vi "Save Data (SubVI).vi"(0 "Time":dbl, 1 "Impedance":dbl[](array[numeric]), 2 "Phase":dbl[](array[numeric]), 3 "error in":errorcluster, 4 "Temperature":dbl, 5 "Byte Stream File in":refnum<file>) -> (6 "error out":errorcluster)   [LabVIEW 2017]
uses:
  GlobalVariables/Delimiter.vi
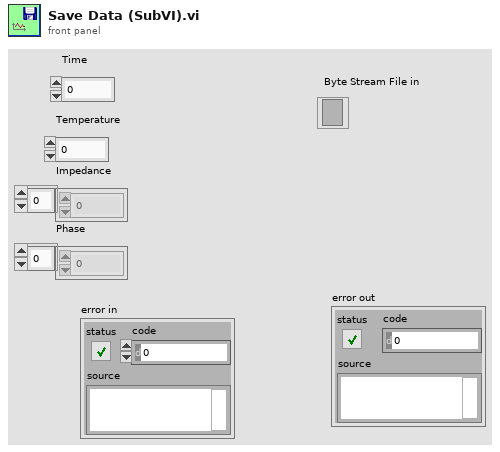
[diagram p1: front panel]
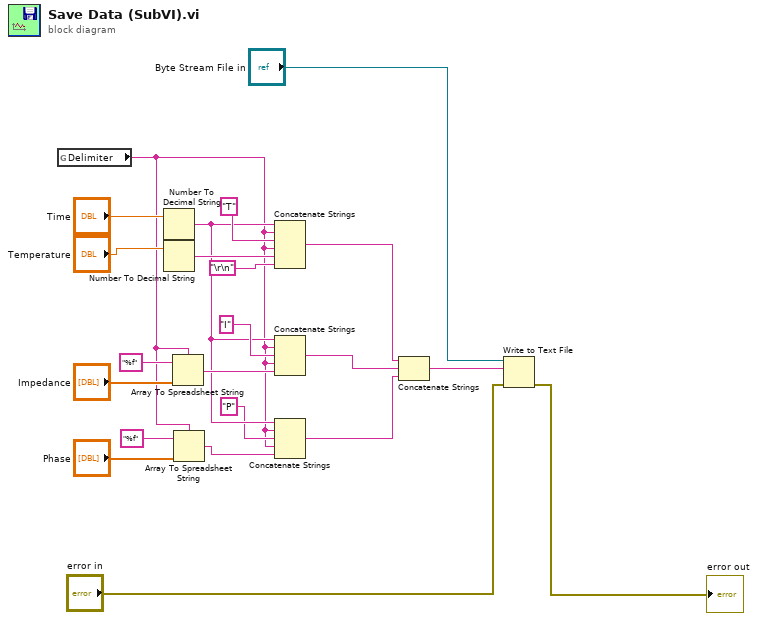
[diagram p0: block diagram]
diagram:
  n1 = global read "Delimiter.vi" "Delimiter"() -> (w9:string)
  n2 = Number To Decimal String(number="Time") -> (decimal integer string=w11:string)  [unwired: 1 in]
  n3 = Number To Decimal String(number="Temperature") -> (decimal integer string=w19:string)  [unwired: 1 in]
  n4 = Array To Spreadsheet String(delimiter (Tab)=w9, array="Impedance", 3:"%f" ("format string")) -> (spreadsheet string=w13:string)
  n5 = Array To Spreadsheet String(delimiter (Tab)=w9, array="Phase", 3:"%f" ("format string")) -> (spreadsheet string=w8:string)
  n6 = Concatenate Strings(w11, w9, "T" ("decimal integer string"), w9, w19, "\r\n") -> (w7:string)
  n7 = Concatenate Strings(w11, w9, "I" ("decimal integer string"), w9, w13) -> (w6:string)
  n8 = Concatenate Strings(w11, w9, "P" ("decimal integer string"), w9, w8) -> (w5:string)
  n9 = Concatenate Strings(w7, w6, w5) -> (w4:string)
  n10 = Write to Text File(file (use dialog)="Byte Stream File in", text=w4, error in="error in") -> (error out=→"error out":errorcluster)  [unwired: 1 in, 2 out]
